vi "EscribirArchivoConfiguracion.vi"(8 "error in":errorcluster, 10 "TipoGenerador":string="Externo", 11 "AjustesPrevios in":refnum<class "AjustesPrevios.lvclass">) -> (0 "error out":errorcluster, 2 "TipoGenerador out":string="Externo", 3 "AjustesPrevios out":refnum<class "AjustesPrevios.lvclass">)   [LabVIEW 2019, in "AjustesPrevios.lvclass"]
uses:
  AjustesPrevios.lvclass
  AjustesPrevios.lvclass/AjustesPrevios.ctl
  <vilib>/Utility/config.llb/Write Key (String).vi
  <vilib>/Utility/config.llb/NI_LVConfig.lvlib
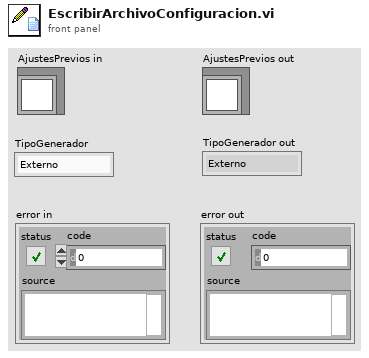
[diagram p1: front panel]
types:
  T1 = typedef "NI_LVConfig.lvlib/Config Data RefNum.ctl" = refnum<k1>
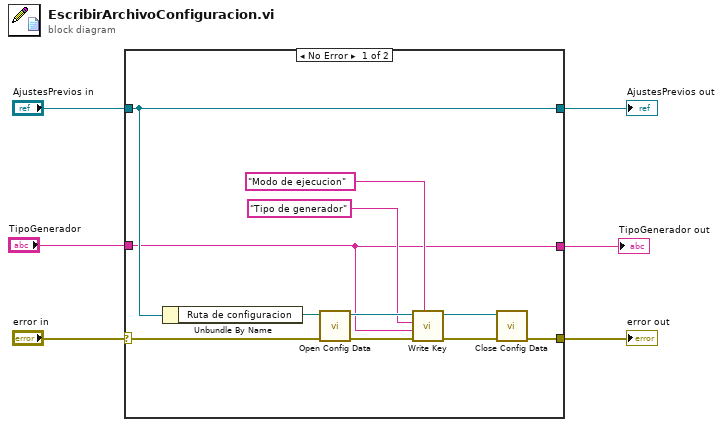
[diagram p0: block diagram]
diagram:
  n1 = case shown="No Error" "error in" {
    selector: "error in" -> [w17 w18]
    tunnel: [w10 w18] -> w4
    tunnel: [w8 w19] -> w6
    tunnel: "AjustesPrevios in" -> [w8 w19]
    tunnel: "TipoGenerador" -> [w7 _]
    tunnel: [w7 _] -> w1
    frame No Error {
      n2 = Unbundle By Name(w8) -> ("Ruta de configuracion"=w16:path)
      n3 = call <vilib>:"Open Config Data.vi"("error in (no error)"=w17, "configuration file path"=w16) -> ("error out"=w15:errorcluster, "refnum"=w14:T1)  [unwired: 7 in, 1 out]
      n4 = call-poly <vilib>:"Write Key.vi"("section"="Modo de ejecucion", "error in (no error)"=w15, "value"=w7, "key"="Tipo de generador", "refnum"=w14) -> ("error out"=w11:errorcluster, "refnum out"=w9:T1)  [unwired: 4 in, 1 out]
      n5 = call <vilib>:"Close Config Data.vi"("error in (no error)"=w11, "refnum"=w9) -> ("error out"=w10:errorcluster)  [unwired: 8 in, 1 out]
    }
    frame Error {
    }
  }
  "AjustesPrevios out" <- w6
  "error out" <- w4
  "TipoGenerador out" <- w1
